vi "Calculate Scope Acquired Time.vi"(0 "Scope Reference Position":dbl, 7 "Acquisition Time":dbl) -> (4 "Scope Acquired Time":dbl)   [LabVIEW 2020, in "LDO Load Transient_AWG.lvlib"]
doc: "This VI returns the scope Acquired time such that all the waveform is fetched\nalong with pretrigger samples because of reference position\nScope Acquired Time = Waveform aqusition time + Time to Pretriggered samples"
uses:
  LDO Load Transient_AWG.lvlib
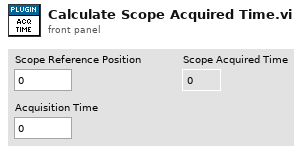
[diagram p1: front panel]
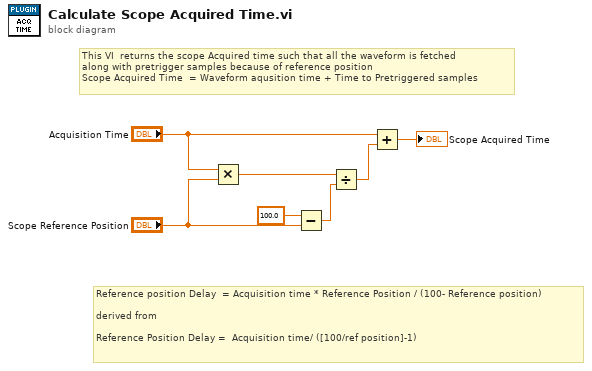
[diagram p0: block diagram]
diagram:
  # "This VI  returns the scope Acquired time such that all the waveform is fetched\nalong with pretrigger samples because of reference position\nScope Acquired Time  = Waveform aqusition time + Time to Pretriggered samples"
  # "Reference position Delay  = Acquisition time * Reference Position / (100- Reference position)\n\nderived from\n\nReference Position Delay =  Acquisition time/ ([100/ref position]-1)"
  n1 = Multiply(x="Acquisition Time", y="Scope Reference Position") -> (x*y=w7:dbl)
  n2 = Subtract(x=100.0, y="Scope Reference Position") -> (x-y=w4:dbl)
  n3 = Divide(x=w7, y=w4) -> (x/y=w2:dbl)
  n4 = Add(x="Acquisition Time", y=w2) -> (x+y=→"Scope Acquired Time":dbl)
